vi "VIPM Request Power Example.vi"() -> ()   [LabVIEW 2024]
uses:
  source/libraries/Request Power.lvlib
panel:
  in  "stop":bool
  in  "keep display on":bool=TRUE
  # "Power Requests are Windows official way of preventing your computer from sleeping and to keep the dispaly on.\nThis is why your display doesn't turn off when you're watching a movie.\nIt is not a mouse wiggler and doesn't require elevated priviledges.\nOnce you stop Requesting Power your computer will go back to however you have the sleep and display settings configured.\n\nCommon LabVIEW tasks that DO NOT prevent the computer from sleeping:\nDAQ\nWriting to a file\nSerial Port access\n\nYou can moniror Windows Power Requests from an command prompt with admin priviledges.\nUse the command \"powercfg -requests\"\n\nHow to use this example\n1: Choose if you want the dispaly to be kept on\n2: Run\n3: Wait until your computer would normally have gone to sleep or the display would turn off.\n4: Push stop\n5: Normal behavoir will be restored"
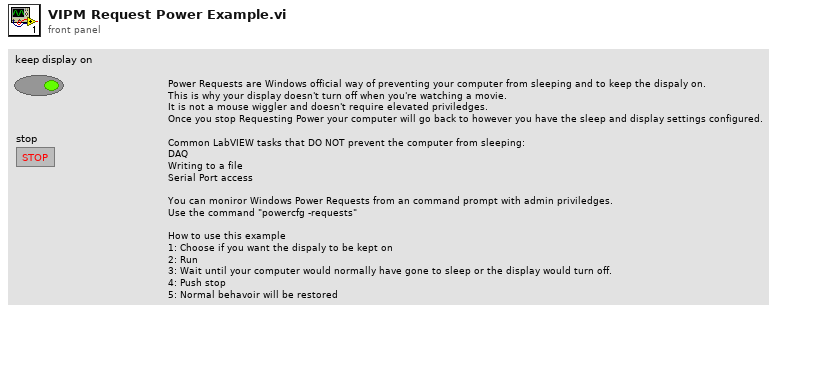
[diagram p1: front panel]
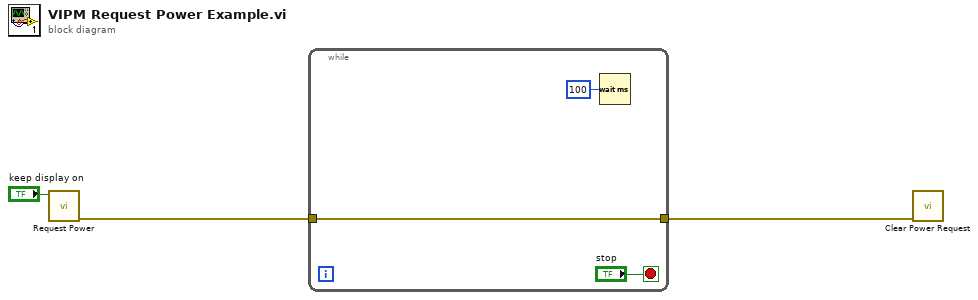
[diagram p0: block diagram]
diagram:
  n1 = call "Request Power.vi"("keep screen on"="keep display on") -> ("error out"=w2:errorcluster)  [unwired: 10 in]
  n2 = while {
    tunnel: w2 -> [w6]
    tunnel: [w6] -> w1
    stop <- "stop" stop-if-true
    n3 = Wait (ms)(milliseconds to wait=u32 100) -> ()  [unwired: 1 out]
  }
  n4 = call "Clear Power Request.vi"("error in (no error)"=w1) -> ()  [unwired: 10 in, 1 out]
